vi "Get Size of Data from TD - Benchmark Set Collection of Fixed-size Type (DBL) - Should Perform in O(1).vi"() -> ()   [LabVIEW 2017, in "Composition.Tests.lvlib"]
uses:
  Composition.Tests.lvlib
  <vilib>/addons/_JKI Toolkits/Caraya/classes/Assert/Assert Less_Variant.vi
  Composition/Composition.lvlib
  <vilib>/addons/_JKI Toolkits/Caraya/classes/Test/Test.lvclass
  <vilib>/addons/_JKI Toolkits/Caraya/classes/Assert/Assert.lvclass
panel:
  out "error out":errorcluster
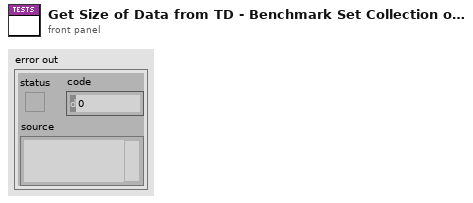
[diagram p1: front panel]
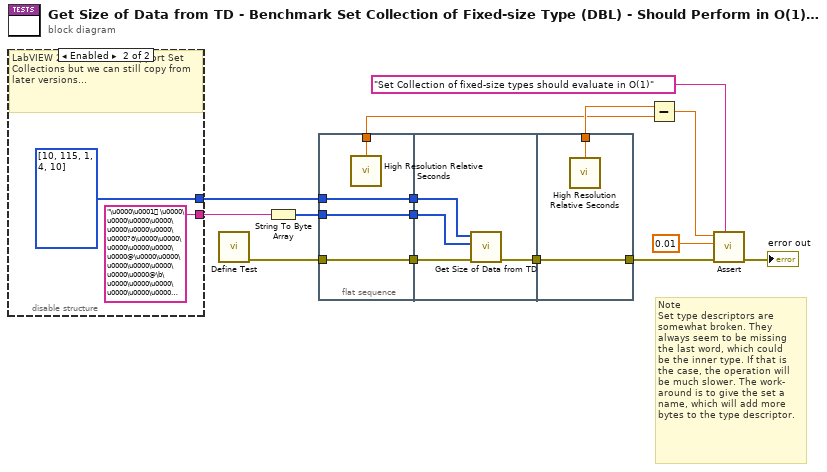
[diagram p0: block diagram]
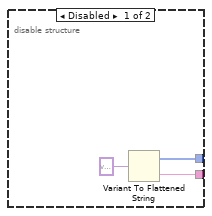
[diagram p2: hidden frame]
diagram:
  # "Note\nSet type descriptors are\nsomewhat broken. They\nalways seem to be missing\nthe last word, which could\nbe the inner type. If that is\nthe case, the operation will\nbe much slower. The work-\naround is to give the set a\nname, which will add more\nbytes to the type descriptor."
  n1 = disable-structure shown="Enabled" {
    disable-tunnel: [w18 "\u0000\u0001 \u0000\u0000\u0000\u0000\u0000\u0000\u0000\u0000?ð\u0000\u0000\u0000\u0000\u0000\u0000@\u0000\u0000\u0000\u0000\u0000\u0000\u0000@\b\u0000\u0000\u0000\u0000\u0000\u0000@\u0010\u0000\u0000\u0000\u0000\u0000\u0000@\u0014\u0000\u0000\u0000\u0000\u0000\u0000@\u0018\u0000\u0000\u0000\u0000\u0000\u0000@\u001c\u0000\u0000\u0000\u0000\u0000\u0000@ \u0000\u0000\u0000\u0000\u0000\u0000@\"\u0000\u0000\u0000\u0000\u0000\u0000@$\u0000\u0000\u0000\u0000\u0000\u0000@&\u0000\u0000\u0000\u0000\u0000\u0000@(\u0000\u0000\u0000\u0000\u0000\u0000@*\u0000\u0000\u0000\u0000\u0000\u0000@,\u0000\u0000\u0000\u0000\u0000\u0000@.\u0000\u0000\u0000\u0000\u0000\u0000@0\u0000\u0000\u0000\u0000\u0000\u0000@1\u0000\u0000\u0000\u0000\u0000\u0000@2\u0000\u0000\u0000\u0000\u0000\u0000@3\u0000\u0000\u0000\u0000\u0000\u0000@4\u0000\u0000\u0000\u0000\u0000\u0000@5\u0000\u0000\u0000\u0000\u0000\u0000@6\u0000\u0000\u0000\u0000\u0000\u0000@7\u0000\u0000\u0000\u0000\u0000\u0000@8\u0000\u0000\u0000\u0000\u0000\u0000@9\u0000\u0000\u0000\u0000\u0000\u0000@:\u0000\u0000\u0000\u0000\u0000\u0000@;\u0000\u0000\u0000\u0000\u0000\u0000@<\u0000\u0000\u0000\u0000\u0000\u0000@=\u0000\u0000\u0000\u0000\u0000\u0000@>\u0000\u0000\u0000\u0000\u0000\u0000@?\u0000\u0000\u0000\u0000\u0000\u0000@@\u0000\u0000\u0000\u0000\u0000\u0000@@\u0000\u0000\u0000\u0000\u0000@A\u0000\u0000\u0000\u0000\u0000\u0000@A\u0000\u0000\u0000\u0000\u0000@B\u0000\u0000\u0000\u0000\u0000\u0000@B\u0000\u0000\u0000\u0000\u0000@C\u0000\u0000\u0000\u0000\u0000\u0000@C\u0000\u0000\u0000\u0000\u0000@D\u0000\u0000\u0000\u0000\u0000\u0000@D\u0000\u0000\u0000\u0000\u0000@E\u0000\u0000\u0000\u0000\u0000\u0000@E\u0000\u0000\u0000\u0000\u0000@F\u0000\u0000\u0000\u0000\u0000\u0000@F\u0000\u0000\u0000\u0000\u0000@G\u0000\u0000\u0000\u0000\u0000\u0000@G\u0000\u0000\u0000\u0000\u0000@H\u0000\u0000\u0000\u0000\u0000\u0000@H\u0000\u0000\u0000\u0000\u0000@I\u0000\u0000\u0000\u0000\u0000\u0000@I\u0000\u0000\u0000\u0000\u0000@J\u0000\u0000\u0000\u0000\u0000\u0000@J\u0000\u0000\u0000\u0000\u0000@K\u0000\u0000\u0000\u0000\u0000\u0000@K\u0000\u0000\u0000\u0000\u0000@L\u0000\u0000\u0000\u0000\u0000\u0000@L\u0000\u0000\u0000\u0000\u0000@M\u0000\u0000\u0000\u0000\u0000\u0000@M\u0000\u0000\u0000\u0000\u0000@N\u0000\u0000\u0000\u0000\u0000\u0000@N\u0000\u0000\u0000\u0000\u0000@O\u0000\u0000\u0000\u0000\u0000\u0000@O\u0000\u0000\u0000\u0000\u0000@P\u0000\u0000\u0000\u0000\u0000\u0000@P@\u0000\u0000\u0000\u0000\u0000@P\u0000\u0000\u0000\u0000\u0000@PÀ\u0000\u0000\u0000\u0000\u0000@Q\u0000\u0000\u0000\u0000\u0000\u0000@Q@\u0000\u0000\u0000\u0000\u0000@Q\u0000\u0000\u0000\u0000\u0000@QÀ\u0000\u0000\u0000\u0000\u0000@R\u0000\u0000\u0000\u0000\u0000\u0000@R@\u0000\u0000\u0000\u0000\u0000@R\u0000..." ("data string")] -> w1
    disable-tunnel: [w16 i16[] [10, 115, 1, 4, 10] ("Type Descriptor")] -> w2
    frame Disabled {
      n2 = Variant To Flattened String(Variant=variant) -> (data string=w18:string, 1:w16:i16[])
    }
    frame Enabled {
      # "LabVIEW 2017 does not support Set Collections but we can still copy from later versions..."
    }
  }
  n3 = call <vilib>:"Define Test.vi"() -> ("error out"=w14:errorcluster)  [unwired: 11 in]
  n4 = String To Byte Array(string=w1) -> (unsigned byte array=w15:u8[])
  n5 = flat-sequence {
    tunnel: w14 -> [w22]
    tunnel: w15 -> [w23]
    tunnel: w2 -> [w24]
    tunnel: [w24] -> w13
    tunnel: [w23] -> w12
    tunnel: [w22] -> w11
    tunnel: [w21] -> w9
    tunnel: w13 -> [w28]
    tunnel: w12 -> [w27]
    tunnel: w11 -> [w26]
    tunnel: [w25] -> w8
    tunnel: [w30] -> w10
    tunnel: [w29] -> w7
    tunnel: w8 -> [w29]
    frame #0 {
      n6 = call <vilib>:"High Resolution Relative Seconds.vi"() -> ("relative seconds"=w21:dbl)
    }
    frame #1 {
      n7 = call "Get Size of Data from TD.vi"("error in (no error)"=w26, "Data String"=w27, "Type Descriptor"=w28) -> ("error out"=w25:errorcluster)  [unwired: 7 in, 1 out]
    }
    frame #2 {
      n8 = call <vilib>:"High Resolution Relative Seconds.vi"() -> ("relative seconds"=w30:dbl)
    }
  }
  n9 = Subtract(x=w10, y=w9) -> (x-y=w6:dbl)
  n10 = call-poly <vilib>:"Assert.vi"("Label"="Set Collection of fixed-size types should evaluate in O(1)", "error in (no error)"=w7, "Y"=0.01 ("x-y"), "X"=w6) -> ("error out"=→"error out":errorcluster)  [unwired: 7 in]
